vi "Parse Parameter Response.vi"(8 "error in":errorcluster, 11 "EF20 in":refnum<class "EF20.lvclass">) -> (0 "error out":errorcluster, 3 "EF20 out":refnum<class "EF20.lvclass">)   [LabVIEW 2018, in "EF20.lvlib" / "EF20.lvclass"]
uses:
  EF20.lvclass
  EF20.lvclass/EF20.ctl
  PPLs/Oven/Oven.lvlibp/Oven.lvclass
  C:/Projects/LabVIEW/PPLs/Oven/Oven.lvlibp/Oven.lvclass
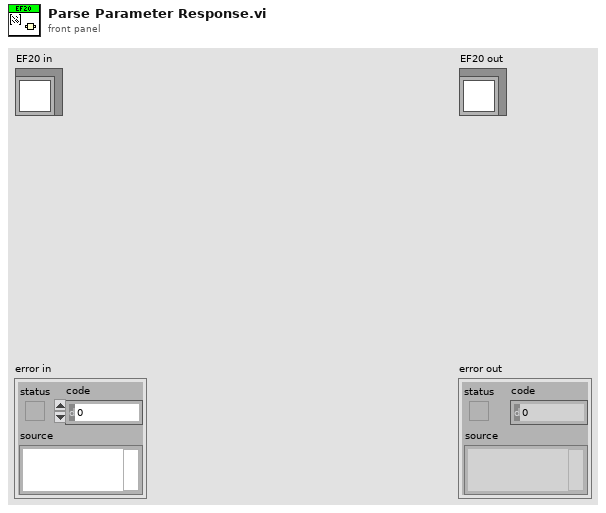
[diagram p1: front panel]
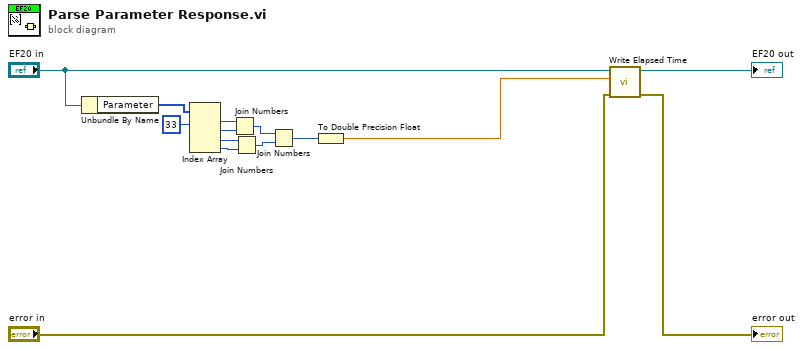
[diagram p0: block diagram]
diagram:
  n1 = Unbundle By Name("EF20 in") -> ("Parameter"=w10:u8[])
  n2 = Index Array(array=w10, index #1=33 ("index")) -> (element #1=w8:u8, element #2=w7:u8, element #3=w6:u8, element #4=w5:u8)  [unwired: 3 in]
  n3 = Join Numbers(hi=w8, lo=w7) -> ((hi.lo)=w4:u16)
  n4 = Join Numbers(hi=w6, lo=w5) -> ((hi.lo)=w3:u16)
  n5 = Join Numbers(hi=w4, lo=w3) -> ((hi.lo)=w2:u32)
  n6 = To Double Precision Float(number=w2) -> (double precision float=w1:dbl)
  n7 = call "Write Elapsed Time.vi"("error in (no error)"="error in", "Elapsed Time"=w1, "Oven in"="EF20 in") -> ("error out"=→"error out":errorcluster, "Oven out"=→"EF20 out":refnum<class "EF20.lvclass">)  [unwired: 7 in]
